vi "Initialize CDO Channel Settings.vi"(11 "array size":i32=8) -> (2 "drive from slot":T1, 3 "channel settings":T2[](array[typedef]))   [LabVIEW 2020, in "Module Test.lvclass"]
uses:
  Module Test Classes/Module Test.lvclass
  Scripting/Modules/Mode Classes/Controls/counter driven output channel settings.ctl
  Scripting/Modules/Channel Classes/Counter Driven Output Channel/Counter Driven State.ctl
  Scripting/Modules/Mode Classes/Counter Driven Output Mode/Drive from Slot.ctl
  Scripting/Modules/Channel Classes/Counter Driven Output Channel/Counter Driven Output Channel.lvclass
  Scripting/Scan Engine Scripting.lvlib
  Scripting/Modules/Mode Classes/Counter Driven Output Mode/Counter Driven Output Mode.lvclass
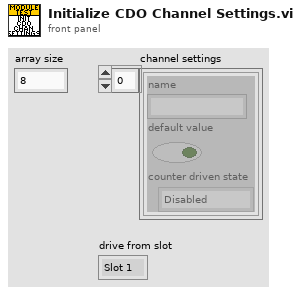
[diagram p1: front panel]
types:
  T1 = typedef "Scan Engine Scripting.lvlib/Counter Driven Output Mode.lvclass/Drive from Slot.ctl" = enum16{"Slot 1", "Slot 2", "Slot 3", "Slot 4", "Slot 5", "Slot 6", "Slot 7", "Slot 8"}
  T2 = typedef "Scan Engine Scripting.lvlib/counter driven output channel settings.ctl" = cluster{"name":string, "default value":bool, "counter driven state":T3}
  T3 = typedef "Scan Engine Scripting.lvlib/Counter Driven Output Channel.lvclass/Counter Driven State.ctl" = enum16{"Disabled", "Enabled"}
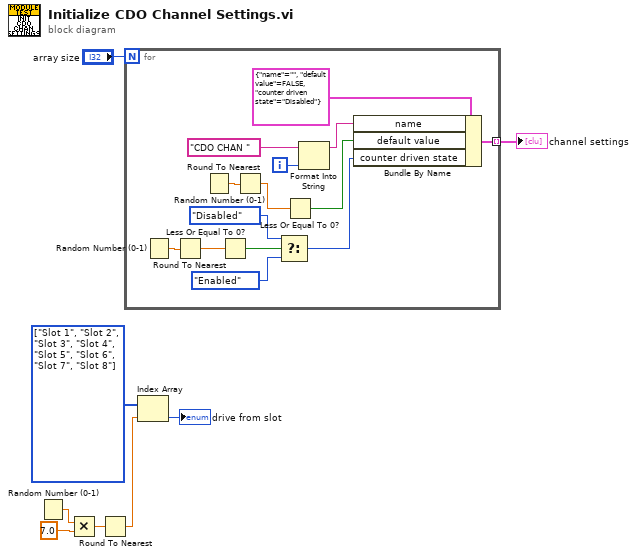
[diagram p0: block diagram]
diagram:
  w2 = T1[] [enum."Slot 1", enum."Slot 2", enum."Slot 3", enum."Slot 4", enum."Slot 5", enum."Slot 6", enum."Slot 7", enum."Slot 8"] items=["Slot 1", "Slot 2", "Slot 3", "Slot 4", "Slot 5", "Slot 6", "Slot 7", "Slot 8"]
  n1 = Random Number (0-1)() -> (number: 0 to 1=w6:dbl)
  n2 = Multiply(x=w6, y=7.0) -> (x*y=w4:dbl)
  n3 = Round To Nearest(number=w4) -> (nearest integer value=w3:dbl)
  n4 = for {
    N: "array size" -> [_]
    tunnel: [w18] -> w7 mode=indexing
    i -> [w11]
    n5 = Random Number (0-1)() -> (number: 0 to 1=w16:dbl)
    n6 = Round To Nearest(number=w16) -> (nearest integer value=w17:dbl)
    n7 = Random Number (0-1)() -> (number: 0 to 1=w22:dbl)
    n8 = Less Or Equal To 0?(x=w17) -> (x <= 0?=w15:bool)
    n9 = Round To Nearest(number=w22) -> (nearest integer value=w21:dbl)
    n10 = Select(t=Counter_Driven_State."Disabled" ("counter driven state"), s=w15, f=Counter_Driven_State."Enabled" ("counter driven state")) -> (s? t:f=w12:T3)
    n11 = Less Or Equal To 0?(x=w21) -> (x <= 0?=w19:bool)
    n12 = Format Into String(initial string="CDO CHAN ", w11) -> (resulting string=w9:string)  [unwired: 2 in, 1 out]
    n13 = Bundle By Name(cluster=T2 {"name"="", "default value"=FALSE, "counter driven state"=enum."Disabled"} ("channel settings"), "name"=w9, "default value"=w19, "counter driven state"=w12) -> (w18:T2)
  }
  "channel settings" <- w7
  n14 = Index Array(array=w2, index=w3) -> (element=→"drive from slot":T1)
